vi "GPIO Timestamp Loop.vi"(0 "fpga interface in":refnum<k20>, 1 "'stop' notifier":refnum<notifier>, 2 "log gpio to disk":bool=TRUE, 5 "tdms file directory":path, 7 "gpio to display":T1[](array[typedef])=[{"GPIO Bank"=enum."Ser0 GPIO Bank", "GPIO Number"=0}], 11 "error in (no error)":errorcluster) -> (6 "gpio timestamps waveform":digitalwaveform[](graph), 8 "error parsing gpio timestamps":bool, 15 "error out":errorcluster)   [LabVIEW 2023, in "GettingStarted_Common_148X_Host.lvlib"]
uses:
  GettingStarted_Common_148X_Host.lvlib
  Types/GPIO Filter.ctl
  <instrlib>/FlexRIO/CSI-2/v2/FPGA/Types/Timestamp ID.ctl
  <instrlib>/FlexRIO/CSI-2/v2/FPGA/NI CSI-2 API FPGA v2.lvlib
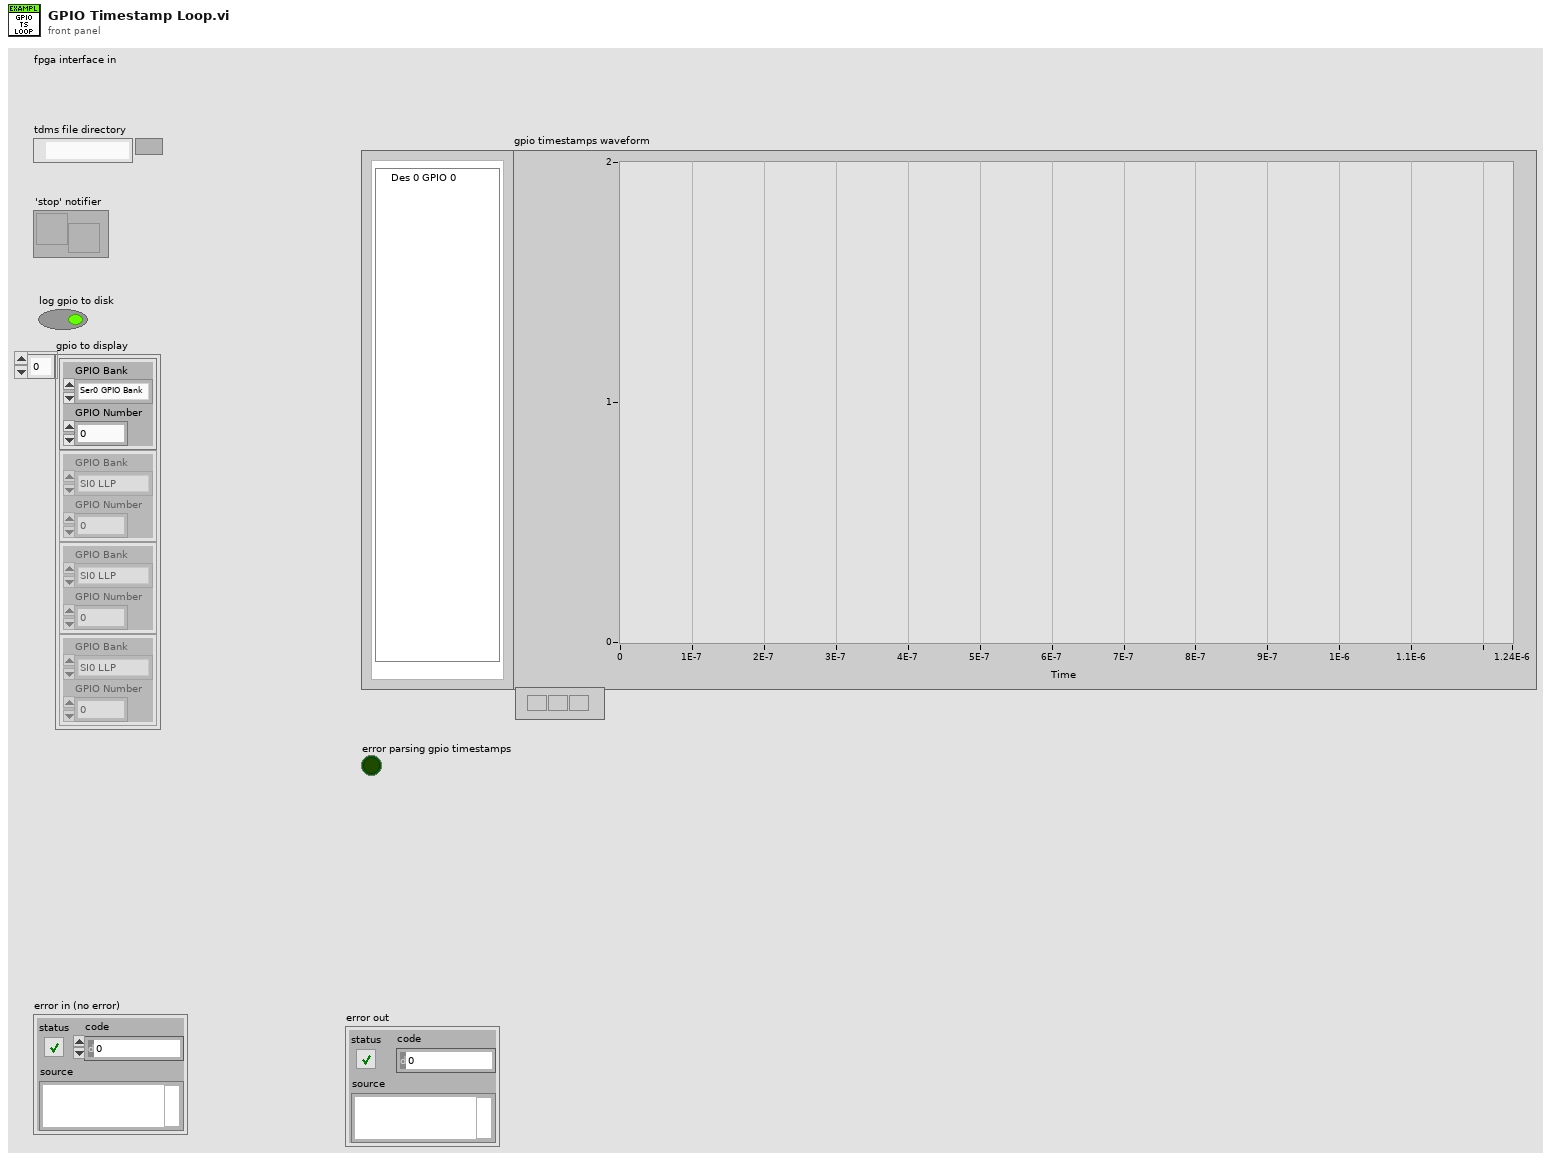
[diagram p1: front panel]
types:
  T1 = typedef "GettingStarted_Common_148X_Host.lvlib/GPIO Filter.ctl" = cluster{"GPIO Bank":T2, "GPIO Number":i32}
  T2 = typedef "NI CSI-2 API FPGA v2.lvlib/Timestamp ID.ctl" = enum8{"SI0 LLP", "SI1 LLP", "SI2 LLP", "SI3 LLP", "SI4 LLP", "SI5 LLP", "SI6 LLP", "SI7 LLP", "SO0 LLP", "SO1 LLP", "SO2 LLP", "SO3 LLP", "SO4 LLP", "SO5 LLP", "SO6 LLP", "SO7 LLP", "Ser0 GPIO Bank", "Ser1 GPIO Bank", "Ser2 GPIO Bank", "Ser3 GPIO Bank", "Ser4 GPIO Bank", "Ser5 GPIO Bank", "Ser6 GPIO Bank", "Ser7 GPIO Bank", "Des0 GPIO Bank", "Des1 GPIO Bank", "Des2 GPIO Bank", "Des3 GPIO Bank", "Des4 GPIO Bank", "Des5 GPIO Bank", "Des6 GPIO Bank", "Des7 GPIO Bank", "User0", "User1", "User2", "User3", "User4", "User5", "User6", "User7", "User8", "User9", "User10", "User11", "User12", "User13", "User14", "User15", "User16", "User17", "User18", "User19", "User20", "User21", "User22", "User23", "User24", "User25", "User26", "User27", "User28", "User29", "User30", "User31"}
  T3 = typedef "NI CSI-2 API Host v2.lvlib/Host GPIO Bank Timestamp.ctl" = cluster{"valid":bool, "count":u64, "id":T2, "gpio bank":T4}
  T4 = typedef "NI CSI-2 API FPGA v2.lvlib/GPIO Bank.ctl" = cluster{"GPIO 0":bool, "GPIO 1":bool, "GPIO 2":bool, "GPIO 3":bool, "GPIO 4":bool, "GPIO 5":bool, "GPIO 6":bool, "GPIO 7":bool, "GPIO 8":bool, "GPIO 9":bool, "GPIO 10":bool}
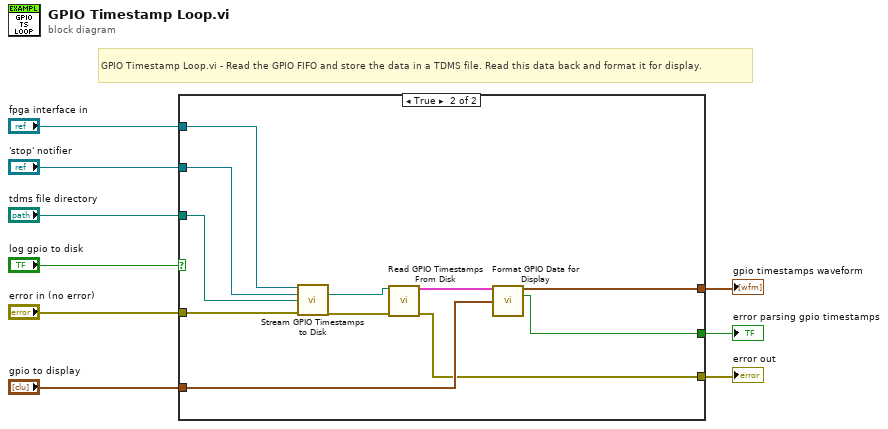
[diagram p0: block diagram]
diagram:
  # "GPIO Timestamp Loop.vi - Read the GPIO FIFO and store the data in a TDMS file. Read this data back and format it for display."
  n1 = case shown="True" "log gpio to disk" {
    tunnel: "error in (no error)" -> [w10 w21]
    tunnel: "fpga interface in" -> [_ w20]
    tunnel: "'stop' notifier" -> [_ w19]
    tunnel: "tdms file directory" -> [_ w18]
    tunnel: "gpio to display" -> [_ w17]
    tunnel: [_ w13] -> w4
    tunnel: [_ w12] -> w3
    tunnel: [w10 w11] -> w2
    frame False {
    }
    frame True {
      n2 = call "Stream GPIO Timestamps to Disk.vi"("fpga interface in"=w20, "'stop' notifier"=w19, "base tdms file path"=w18, "error in (no error)"=w21) -> ("file path out"=w16:path, "error out"=w15:errorcluster)  [unwired: 8 in, 2 out]
      n3 = call "Read GPIO Timestamps From Disk.vi"("file path"=w16, "error in (no error)"=w15) -> ("gpio timestamps"=w14:T3[], "error out"=w11:errorcluster)  [unwired: 12 in]
      n4 = call "Format GPIO Data for Display.vi"("gpio timestamps"=w14, "gpio to display"=w17) -> ("gpio timestamps waveform"=w12:digitalwaveform[], "error parsing timestamps"=w13:bool)  [unwired: 12 in]
    }
  }
  "error out" <- w2
  "gpio timestamps waveform" <- w3
  "error parsing gpio timestamps" <- w4
